vi "MoveAbsolute.vi"(8 "error in (no error)":errorcluster, 10 "Move Abs Value":dbl, 11 "ThorlabsLabJack in":refnum<class "ThorlabsLabJack.lvclass">) -> (0 "error out":errorcluster, 3 "ThorlabsLabJack out":refnum<class "ThorlabsLabJack.lvclass">)   [LabVIEW 2018, in "ThorlabsLabJack.lvlib" / "ThorlabsLabJack.lvclass"]
uses:
  ThorlabsLabJack.lvclass
  ThorlabsLabJack.lvclass/ThorlabsLabJack.ctl
  C:/AME Test Engineering/LabVIEW/PPLs/Axis/Thorlabs/Thorlabs.MotionControl.IntegratedStepperMotorsCLI.dll
  PPLs/Axis/Thorlabs/Thorlabs.MotionControl.IntegratedStepperMotorsCLI.dll
  a1f4e168-4b5a-4ae4-ba4d-f49253613271.vi
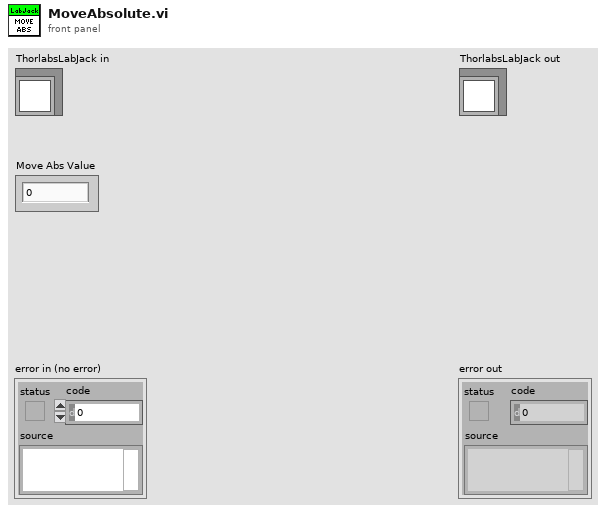
[diagram p1: front panel]
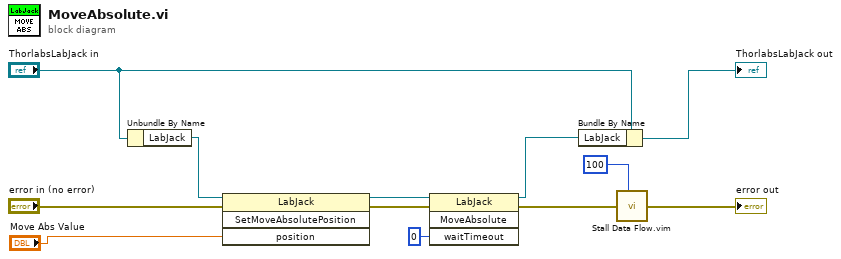
[diagram p0: block diagram]
diagram:
  n1 = Unbundle By Name("ThorlabsLabJack in") -> ("LabJack"=w9:refnum<k24>)
  n2 = invoke class="LabJack" method="SetMoveAbsolutePosition"(reference=w9, error in="error in (no error)", "position"="Move Abs Value") -> (reference out=w7:refnum<k24>, error out=w6:errorcluster)  [unwired: 1 in, 2 out]
  n3 = invoke class="LabJack" method="MoveAbsolute"(reference=w7, error in=w6, "waitTimeout"=0) -> (reference out=w4:refnum<k24>, error out=w3:errorcluster)  [unwired: 1 in, 2 out]
  n4 = Bundle By Name(cluster="ThorlabsLabJack in", "LabJack"=w4) -> (→"ThorlabsLabJack out":refnum<class "ThorlabsLabJack.lvclass">)
  n5 = call "Stall Data Flow.vim"("value in"=w3, "milliseconds to wait"=u32 100) -> ("value out"=→"error out":errorcluster)  [unwired: 1 out]
